vi "FPGA.vi"() -> ()   [LabVIEW 2020]
uses:
  <vilib>/Platform/TimedLoop/XDataNode/timing_clust.ctl
  <vilib>/Platform/TimedLoop/XDataNode/nitl_modes.ctl
  <vilib>/Platform/TimedLoop/XDataNode/wakeup.ctl
  <vilib>/rvi/Analysis/measure/FFT/simModelSupport/niFPGA FFT Sim Properties.ctl
  <vilib>/rvi/Analysis/measure/FFT/simModelSupport/niFPGA FFT Sim Types.ctl
  <vilib>/rvi/Analysis/measure/FFT/simModelSupport/niFpgaFFTSimArithmeticProperties.ctl
  <vilib>/rvi/Analysis/measure/FFT/simModelSupport/niFpgaFFTSimDfxp.ctl
  <vilib>/fxp/LVFixedPointQuantizationPolicyTypeDef.ctl
  <vilib>/rvi/DataTransferAndStorage/Container/Common/niFpgaContainerGetUniqueNameForEmu.vi
  <vilib>/rvi/DataTransferAndStorage/Container/Common/niFpgaContainerSetEmuInfo.vi
  <vilib>/rvi/eio/common/nirviEmuReportErrorAndStop.vi
  <vilib>/rvi/eio/common/nirviEmuTemplateMethod_errors.vi
  <vilib>/rvi/DataTransferAndStorage/Container/Common/niFpgaContainerExecOnDevCompGetState.vi
  <vilib>/rvi/Emulation/niFpgaEmulationIsFPGAContextNoSignature.vi
  <vilib>/rvi/Emulation/niFpgaSctlEmulationGetInTimedLoop.vi
  <vilib>/rvi/errors/niFpgaSetErrorForExecOnDevCompSimple.vi
  <vilib>/rvi/FIFO/Fifo_Resource/nirvififoEmulationSetSize.vi
  <vilib>/rvi/FIFO/Fifo_Resource/nirviFifoEmulationQueueMgr.vi
  <instcachedir>/0/nirviFifoEmulationQueueMgr_E5CAEC123FF24DC58D834DCA3CDAA9B5.lvgen/nirviFifoEmulationQueueMgr_E5CAEC123FF24DC58D834DCA3CDAA9B5_003.vi
  <vilib>/rvi/FIFO/Fifo_Resource/nirvififoEmulationDetermineInputValidOut.vi
  <vilib>/rvi/FIFO/Fifo_Resource/nirvififoEmulationCreateLock.vi
  <vilib>/rvi/Emulation/niFpgaProcessEmulError.vi
  <vilib>/rvi/FIFO/Fifo_Resource/nirvififoEmulationObtainLock.vi
  <vilib>/rvi/FIFO/Fifo_Resource/nirvififoEmulationReleaseLock.vi
  <vilib>/rvi/occurrence/nirviWaitOnOccurrenceBase.vi
  <vilib>/rvi/errors/nirviReportUnexpectedCaseInternalError.vi
  <vilib>/rvi/errors/nirviReportUnexpectedCaseInternalError (U32).vi
  <vilib>/Utility/error.llb/Clear Errors.vi
  <vilib>/rvi/interface/RandomDataEmulation/niFpgaRandomDataHandleErrors.vi
  <vilib>/rvi/Emulation/niFpgaEmulationReportErrorSimple.vi
  <vilib>/rvi/Emulation/niFpgaGetClockAttributes.vi
  <vilib>/rvi/Emulation/niFpgaCriticalErrorInLSC.vi
  <vilib>/rvi/Analysis/measure/FFT/simModelSupport/niFpgaFFTSimModelCore.vi
  <vilib>/rvi/LocalResourceManager/LocalResourceManager.xnode
  <vilib>/eio/EIONode/EIONode.xnode
  <vilib>/rvi/DataTransferAndStorage/Container/XNode/niFpgaContainer.xnode
  <vilib>/rvi/FIFO/Fifo_Resource/niFpgaFifoEmulationRefIn.vi
  <vilib>/Platform/TimedLoop/XDataNode/XDataNode.xnode
  <vilib>/rvi/interface/RandomDataEmulation/nirviRandomDataFpgaReadWriteTemplate.vi
  <vilib>/rvi/Analysis/measure/FFT/XNode/niFpgaFFT.xnode
  <vilib>/rvi/FXPMathLib/FxpInterpret/XNode/nifxpmath_Interpret.xnode
  <vilib>/Platform/TimedLoop/XDataNode/XDNodeRunTimeDep.lvlib
panel:
  in  "Rate (uSec)":u32 caption="Count(uSec)"
  out "Timed Out? FIFO out index 2":bool
  out "Timed Out? FIFO out IMG 2":bool
  out "Timed Out? FIFO out REAL 2":bool
  out "Timed Out? FIFO in IMG":bool
  out "Timed Out? FIFO in REAL":bool
  out "Timed Out? FIFO out REAL":bool
  out "Timed Out? FIFO out IMG":bool
  out "Timed Out? FIFO out index":bool
  in  "FFT loop iterations":i32
  in  "auto stop":bool
  in  "Loop number":i32
  out "AI Timed Out?":bool
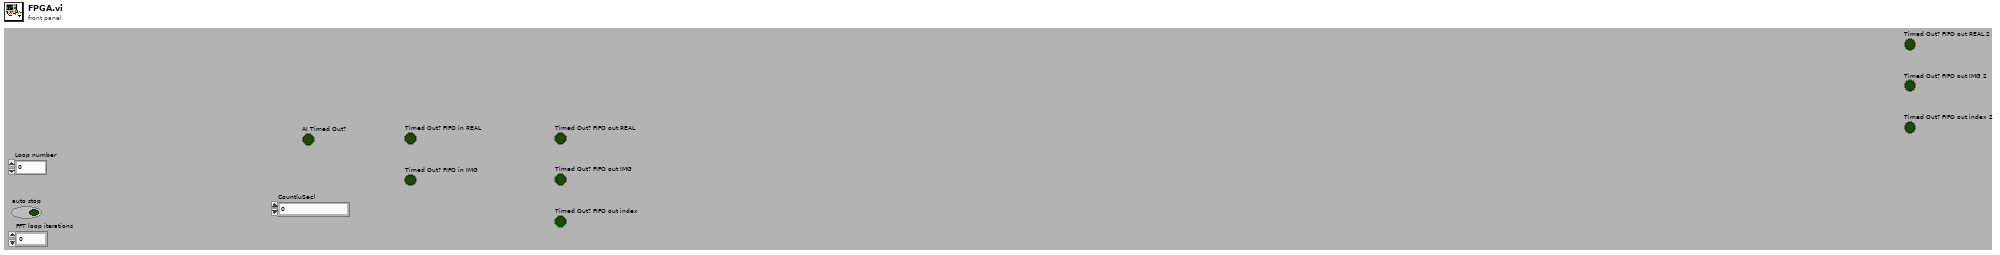
[diagram p1: front panel]
types:
  T1 = typedef "XDNodeRunTimeDep.lvlib/timing_clust.ctl" = cluster{"Expected End [f-1]":u64, "Actual End [f-1]":u64, "Finished Late? [f-1]":bool, "Expected End [i-1]":u64, "Actual End [i-1]":u64, "Finished Late? [i-1]":bool, "Expected Start [i]":u64, "Actual Start [i]":u64, "Expected Start [f]":u64, "Actual Start [f]":u64, "Source Name":string, "Structure Name":string, "Period":i64, "Deadline":i64, "Offset":i64, "Start":i64, "Priority":i32, "Timeout":i32, "Mode":T2, "Wakeup Reason":T3, "Error":errorcluster, "Source Type":string, "Secondary Source Type":string, "Global End Time":u64, "Global Start Time":u64, "Frame Duration":u64, "Iteration Duration":u64, "Assigned CPU":i32, "I/O Scan Engine Mode":u32}
  T2 = typedef "XDNodeRunTimeDep.lvlib/nitl_modes.ctl" = enum32{"No Change", "Process missed periods, maintain original phase", "Discard missed periods, maintain original phase", "Process missed periods, ignore original phase", "Discard missed periods, ignore original phase"}
  T3 = typedef "XDNodeRunTimeDep.lvlib/wakeup.ctl" = enum32{"Normal", "Aborted", "Asynchronous wakeup", "Timing source error", "Timed loop error", "Timeout"}
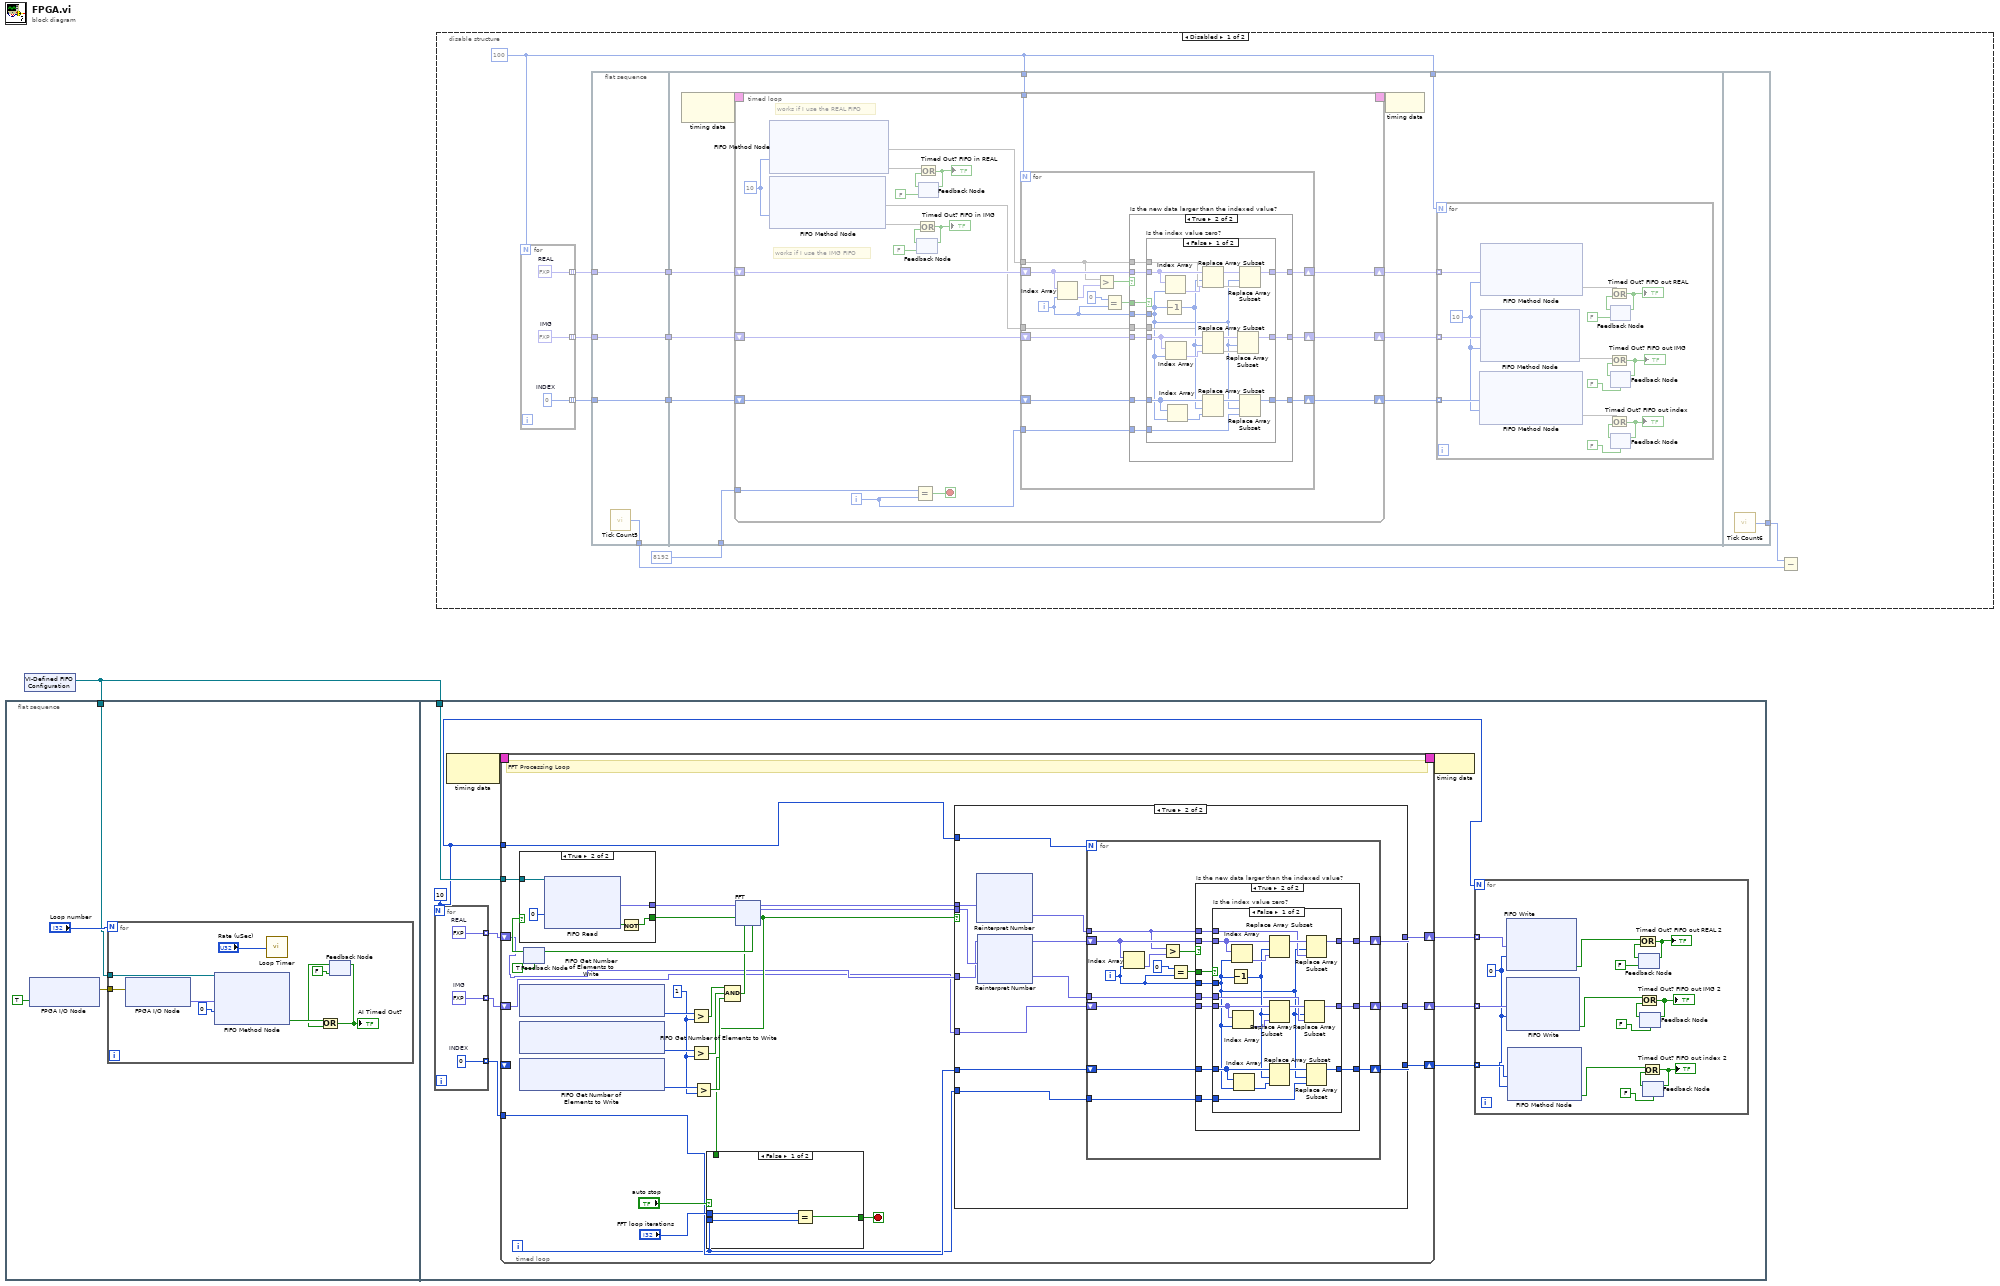
[diagram p0: block diagram]
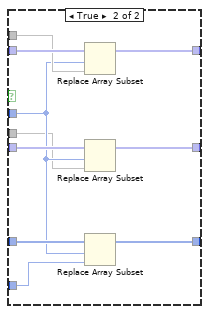
[diagram p3: hidden frame]
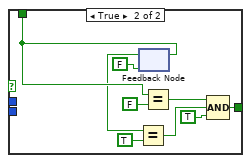
[diagram p5: hidden frame]
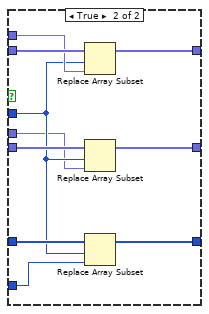
[diagram p8: hidden frame]
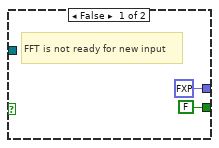
[diagram p9: hidden frame]
diagram:
  n1 = flat-sequence {
    tunnel: w1 -> [w4]
    tunnel: w1 -> [w22]
    frame #0 {
      n2 = xnode "FPGA I/O Node"("Mod1/Start"=TRUE) -> ("error out"=w2:errorcluster)  [unwired: 2 in, 1 out]
      n3 = for {
        N: "Loop number" -> [_]
        tunnel: w4 -> [w14]
        tunnel: w2 -> [w7]
        n4 = xnode "FPGA I/O Node"("error in"=w7) -> ("Mod1/AI0"=w8:fxp<+/-,24,7>)  [unwired: 1 in, 2 out]
        n5 = xnode ("FIFO Method Node")("Element"=w8, "Timeout"=0, "FIFO In"=w14) -> ("Timed Out?"=w12:bool)  [unwired: 1 in, 2 out]
        n6 = call "Loop Timer"("Count(uSec)"="Rate (uSec)") -> ()  [unwired: 1 out]
        n7 = feedback #1(FALSE) -> (w11:bool)
        n8 = Or(x=w12, y=w11) -> (x .or. y?=w10:bool)
        "AI Timed Out?" <- w10
        n9 = feedback-in #1(w10) -> ()
      }
    }
    frame #1 {
      w15 = 10
      n10 = for {
        N: w15 -> [_]
        tunnel: [w43] -> w21 mode=indexing
        tunnel: [w42] -> w19 mode=indexing
        tunnel: [w41] -> w20 mode=indexing
        w41 = fxp<+/-,32,21> 0.0  # IMG
        w42 = 0  # INDEX
        w43 = fxp<+/-,32,21> 0.0  # REAL
      }
      n11 = node-c288() -> (w24:T1)  [unwired: 1 in]
      n12 = timed-loop {
        timing: w24 -> [_]
        timing-out: [_] -> w23
        tunnel: w22 -> [w68]
        tunnel: w19 -> [w49]
        tunnel: w15 -> [w44]
        shift-right: [w45] -> w16
        shift-left: _ -> [_]
        shift-right: [w46] -> w18
        shift-left: w20 -> [w50]
        shift-right: [w47] -> w17
        shift-left: w21 -> [w51]
        i -> [w48]
        stop <- w56 stop-if-true
        w62 = u32 1 ("y")
        # "FFT Processing Loop"
        n13 = xnode ("FIFO Get Number of Elements to Write")() -> ("Number of Elements to Write"=w65:u32)  [unwired: 1 in, 1 out]
        n14 = xnode ("FIFO Get Number of Elements to Write")() -> ("Number of Elements to Write"=w64:u32)  [unwired: 1 in, 1 out]
        n15 = xnode ("FIFO Get Number of Elements to Write")() -> ("Number of Elements to Write"=w63:u32)  [unwired: 1 in, 1 out]
        n16 = feedback #2(TRUE ("ready for input")) -> (w71:bool)
        n17 = case shown="True" w71 {
          tunnel: [FALSE w185] -> w58
          tunnel: [fxp<+/-,16,5> 0.0 ("Element") w186] -> w70
          tunnel: w68 -> [_ w182]
          frame False {
            # "FFT is not ready for new input"
          }
          frame True {
            n18 = xnode ("FIFO Read")("Timeout"=0, "FIFO In"=w182) -> ("Element"=w186:fxp<+/-,24,7>, "Timed Out?"=w184:bool)  [unwired: 1 out]
            n19 = Not(x=w184) -> (.not. x?=w185:bool)
          }
        }
        n20 = Greater?(x=w65, y=w62) -> (0:w61:bool)
        n21 = Greater?(x=w64, y=w62) -> (0:w60:bool)
        n22 = Greater?(x=w63, y=w62) -> (0:w59:bool)
        n23 = Compound Arithmetic op=AND(w61, w60, w59) -> (w57:bool)
        n24 = xnode "FFT"("real data in"=w70, "input valid"=w58, "ready for output"=w57) -> ("ready for input"=w69:bool, "real data out"=w67:fxp<+/-,32,15>, "imaginary data out"=w55:fxp<+/-,32,15>, "output valid"=w52:bool)  [unwired: 2 in, 1 out]
        n25 = feedback-in #2(w69) -> ()
        n26 = case shown="False" "auto stop" {
          tunnel: w52 -> [_ w82]
          tunnel: [w72 w75] -> w56
          tunnel: w48 -> [w74 _]
          tunnel: "FFT loop iterations" -> [w73 _]
          frame False {
            n27 = Equal?(x=w73, y=w74) -> (x = y?=w72:bool)
          }
          frame True {
            n28 = feedback #3(FALSE) -> (w79:bool)
            n29 = Equal?(x=w79, y=TRUE) -> (x = y?=w77:bool)
            n30 = feedback-in #3(w82) -> ()
            n31 = Equal?(x=w82, y=FALSE) -> (x = y?=w78:bool)
            n32 = Compound Arithmetic op=AND(w78, w77, TRUE ("value")) -> (w75:bool)
          }
        }
        n33 = case shown="True" w52 {
          tunnel: w67 -> [_ w124]
          tunnel: w55 -> [_ w123]
          tunnel: w51 -> [w112 w120]
          tunnel: w50 -> [w111 w119]
          tunnel: w49 -> [w110 w118]
          tunnel: w48 -> [_ w117]
          tunnel: [w112 w116] -> w47
          tunnel: [w111 w115] -> w46
          tunnel: [w110 w114] -> w45
          tunnel: w44 -> [_ w113]
          frame False {
          }
          frame True {
            n34 = xnode "Reinterpret Number"("x"=w124) -> ("y"=w122:fxp<+/-,32,21>)
            n35 = xnode "Reinterpret Number"("x"=w123) -> ("y"=w121:fxp<+/-,32,21>)
            n36 = for {
              N: w113 -> [_]
              tunnel: w122 -> [w135]
              shift-right: [w134] -> w116
              shift-left: w120 -> [w136]
              tunnel: w117 -> [w132]
              shift-right: [w130] -> w114
              shift-left: w118 -> [w131]
              shift-right: [w127] -> w115
              shift-left: w119 -> [w126]
              tunnel: w121 -> [w125]
              i -> [w133]
              n37 = Index Array(array=w136, index=w133) -> (element=w138:fxp<+/-,32,21>)
              n38 = Greater?(x=w135, y=w138) -> (0:w137:bool)
              n39 = Equal?(x=0, y=w133) -> (x = y?=w128:bool)
              n40 = case "Is the new data larger than the indexed value?" shown="True" w137 {
                tunnel: w136 -> [w141 w151]
                tunnel: w128 -> [_ w152]
                tunnel: w135 -> [_ w150]
                tunnel: w133 -> [_ w149]
                tunnel: [w141 w148] -> w134
                tunnel: w132 -> [_ w147]
                tunnel: w131 -> [w140 w146]
                tunnel: [w140 w145] -> w130
                tunnel: [w139 w144] -> w127
                tunnel: w126 -> [w139 w143]
                tunnel: w125 -> [_ w142]
                frame False {
                }
                frame True {
                  n41 = case "Is the index value zero?" shown="False" w152 {
                    tunnel: w151 -> [w169 w179]
                    tunnel: w150 -> [w166 w178]
                    tunnel: w149 -> [w153 w172]
                    tunnel: [w165 w177] -> w148
                    tunnel: w147 -> [w160 w176]
                    tunnel: w146 -> [w162 w175]
                    tunnel: [w161 w174] -> w145
                    tunnel: [w155 w170] -> w144
                    tunnel: w143 -> [w159 w173]
                    tunnel: w142 -> [w154 w171]
                    frame False {
                      n42 = Decrement(x=w153) -> (x-1=w157:i32)
                      n43 = Index Array(array=w169, index=w153) -> (element=w168:fxp<+/-,32,21>)
                      n44 = Index Array(array=w159, index=w153) -> (element=w158:fxp<+/-,32,21>)
                      n45 = Index Array(array=w162, index=w153) -> (element=w164:i32)
                      n46 = Replace Array Subset(array=w169, new element=w168, index=w157) -> (w167:fxp<+/-,32,21>[])
                      n47 = Replace Array Subset(array=w159, new element=w158, index=w157) -> (w156:fxp<+/-,32,21>[])
                      n48 = Replace Array Subset(array=w162, new element=w164, index=w157) -> (w163:i32[])
                      n49 = Replace Array Subset(array=w156, new element=w154, index=w153) -> (w155:fxp<+/-,32,21>[])
                      n50 = Replace Array Subset(array=w167, new element=w166, index=w153) -> (w165:fxp<+/-,32,21>[])
                      n51 = Replace Array Subset(array=w163, new element=w160, index=w153) -> (w161:i32[])
                    }
                    frame True {
                      n52 = Replace Array Subset(array=w179, new element=w178, index=w172) -> (w177:fxp<+/-,32,21>[])
                      n53 = Replace Array Subset(array=w173, new element=w171, index=w172) -> (w170:fxp<+/-,32,21>[])
                      n54 = Replace Array Subset(array=w175, new element=w176, index=w172) -> (w174:i32[])
                    }
                  }
                }
              }
            }
          }
        }
      }
      n55 = node-c288(w23) -> ()
      n56 = for {
        N: w15 -> [_]
        tunnel: w18 -> [w40] mode=indexing
        tunnel: w17 -> [w39] mode=indexing
        tunnel: w16 -> [w29] mode=indexing
        w28 = 0 ("Timeout")
        n57 = xnode ("FIFO Write")("Element"=w39, "Timeout"=w28) -> ("Timed Out?"=w25:bool)  [unwired: 1 in, 1 out]
        n58 = xnode ("FIFO Write")("Element"=w40, "Timeout"=w28) -> ("Timed Out?"=w26:bool)  [unwired: 1 in, 1 out]
        n59 = xnode ("FIFO Method Node")("Element"=w29, "Timeout"=w28) -> ("Timed Out?"=w27:bool)  [unwired: 1 in, 1 out]
        n60 = feedback #4(FALSE) -> (w36:bool)
        n61 = Or(x=w25, y=w36) -> (x .or. y?=w37:bool)
        "Timed Out? FIFO out REAL 2" <- w37
        n62 = feedback-in #4(w37) -> ()
        n63 = feedback #5(FALSE) -> (w35:bool)
        n64 = Or(x=w26, y=w35) -> (x .or. y?=w34:bool)
        "Timed Out? FIFO out IMG 2" <- w34
        n65 = feedback-in #5(w34) -> ()
        n66 = feedback #6(FALSE) -> (w32:bool)
        n67 = Or(x=w27, y=w32) -> (x .or. y?=w31:bool)
        "Timed Out? FIFO out index 2" <- w31
        n68 = feedback-in #6(w31) -> ()
      }
    }
  }
  n69 = xnode "VI-Defined FIFO Configuration"() -> ("FIFO Out"=w1:refnum<k21>)
  n70 = disable-structure shown="Disabled" {
    frame Disabled {
      w192 = 100
      n71 = for {
        N: w192 -> [_]
        tunnel: [w203] -> w194 mode=indexing
        tunnel: [w202] -> w195 mode=indexing
        tunnel: [w201] -> w191 mode=indexing
        w201 = fxp<+/-,32,21> 0.0  # IMG
        w202 = 0  # INDEX
        w203 = fxp<+/-,32,21> 0.0  # REAL
      }
      n72 = flat-sequence {
        tunnel: [w207] -> w196
        tunnel: [w206] -> w200
        tunnel: w195 -> [w206]
        tunnel: [w205] -> w199
        tunnel: w194 -> [w205]
        tunnel: [w204] -> w198
        tunnel: w191 -> [w204]
        tunnel: w200 -> [w218]
        tunnel: w199 -> [w217]
        tunnel: 8192 ("samples") -> [w215]
        tunnel: w192 -> [w216]
        tunnel: w192 -> [w212]
        tunnel: w198 -> [w208]
        tunnel: [w315] -> w197
        frame #0 {
          n73 = call "Tick Count5"() -> ("Tick Count(uSec)"=w207:u32)
        }
        frame #1 {
          n74 = node-c288() -> (w214:T1)  [unwired: 1 in]
          n75 = timed-loop {
            shift-right: [w254] -> w210
            shift-left: w217 -> [w255]
            shift-right: [w253] -> w211
            shift-left: w218 -> [w252]
            tunnel: w216 -> [w251]
            tunnel: w215 -> [w249]
            timing: w214 -> [_]
            timing-out: [_] -> w213
            shift-right: [w247] -> w209
            shift-left: w208 -> [w246]
            i -> [w250]
            stop <- w248 stop-if-true
            w245 = 10 ("Timeout")
            # "works if I use the REAL FIFO"
            # "works if I use the IMG FIFO"
            n76 = xnode ("FIFO Method Node")("Timeout"=w245) -> ("Element"=w243, "Timed Out?"=w235)  [unwired: 1 in, 1 out]
            n77 = xnode ("FIFO Method Node")("Timeout"=w245) -> ("Element"=w244, "Timed Out?"=w239)  [unwired: 1 in, 1 out]
            n78 = Equal?(x=w249, y=w250) -> (x = y?=w248:bool)
            n79 = feedback #7(FALSE) -> (w240:bool)
            n80 = Or(x=w239, y=w240) -> (x .or. y?=w241:bool)
            "Timed Out? FIFO in IMG" <- w241
            n81 = feedback-in #7(w241) -> ()
            n82 = feedback #8(FALSE) -> (w236:bool)
            n83 = Or(x=w235, y=w236) -> (x .or. y?=w237:bool)
            "Timed Out? FIFO in REAL" <- w237
            n84 = feedback-in #8(w237) -> ()
            n85 = for {
              N: w251 -> [_]
              tunnel: w243 -> [w266]
              shift-right: [w265] -> w254
              shift-left: w255 -> [w267]
              tunnel: w250 -> [w263]
              shift-right: [w261] -> w253
              shift-left: w252 -> [w262]
              shift-right: [w258] -> w247
              shift-left: w246 -> [w257]
              tunnel: w244 -> [w256]
              i -> [w264]
              n86 = Index Array(array=w267, index=w264) -> (element=w269:fxp<+/-,32,21>)
              n87 = Greater?(x=w266, y=w269) -> (0:w268:bool)
              n88 = Equal?(x=0, y=w264) -> (x = y?=w259:bool)
              n89 = case "Is the new data larger than the indexed value?" shown="True" w268 {
                tunnel: w267 -> [w272 w282]
                tunnel: w259 -> [_ w283]
                tunnel: w266 -> [_ w281]
                tunnel: w264 -> [_ w280]
                tunnel: [w272 w279] -> w265
                tunnel: w263 -> [_ w278]
                tunnel: w262 -> [w271 w277]
                tunnel: [w271 w276] -> w261
                tunnel: [w270 w275] -> w258
                tunnel: w257 -> [w270 w274]
                tunnel: w256 -> [_ w273]
                frame False {
                }
                frame True {
                  n90 = case "Is the index value zero?" shown="False" w283 {
                    tunnel: w282 -> [w300 w310]
                    tunnel: w281 -> [w297 w309]
                    tunnel: w280 -> [w284 w303]
                    tunnel: [w296 w308] -> w279
                    tunnel: w278 -> [w291 w307]
                    tunnel: w277 -> [w293 w306]
                    tunnel: [w292 w305] -> w276
                    tunnel: [w286 w301] -> w275
                    tunnel: w274 -> [w290 w304]
                    tunnel: w273 -> [w285 w302]
                    frame False {
                      n91 = Decrement(x=w284) -> (x-1=w288:i32)
                      n92 = Index Array(array=w300, index=w284) -> (element=w299:fxp<+/-,32,21>)
                      n93 = Index Array(array=w290, index=w284) -> (element=w289:fxp<+/-,32,21>)
                      n94 = Index Array(array=w293, index=w284) -> (element=w295:i32)
                      n95 = Replace Array Subset(array=w300, new element=w299, index=w288) -> (w298:fxp<+/-,32,21>[])
                      n96 = Replace Array Subset(array=w290, new element=w289, index=w288) -> (w287:fxp<+/-,32,21>[])
                      n97 = Replace Array Subset(array=w293, new element=w295, index=w288) -> (w294:i32[])
                      n98 = Replace Array Subset(array=w287, new element=w285, index=w284) -> (w286:fxp<+/-,32,21>[])
                      n99 = Replace Array Subset(array=w298, new element=w297, index=w284) -> (w296:fxp<+/-,32,21>[])
                      n100 = Replace Array Subset(array=w294, new element=w291, index=w284) -> (w292:i32[])
                    }
                    frame True {
                      n101 = Replace Array Subset(array=w310, new element=w309, index=w303) -> (w308:fxp<+/-,32,21>[])
                      n102 = Replace Array Subset(array=w304, new element=w302, index=w303) -> (w301:fxp<+/-,32,21>[])
                      n103 = Replace Array Subset(array=w306, new element=w307, index=w303) -> (w305:i32[])
                    }
                  }
                }
              }
            }
          }
          n104 = node-c288(w213) -> ()
          n105 = for {
            N: w212 -> [_]
            tunnel: w211 -> [w234] mode=indexing
            tunnel: w210 -> [w233] mode=indexing
            tunnel: w209 -> [w232] mode=indexing
            w231 = 10 ("Timeout")
            n106 = xnode ("FIFO Method Node")("Element"=w234, "Timeout"=w231) -> ("Timed Out?"=w219)  [unwired: 1 in, 1 out]
            n107 = xnode ("FIFO Method Node")("Element"=w233, "Timeout"=w231) -> ("Timed Out?"=w227)  [unwired: 1 in, 1 out]
            n108 = xnode ("FIFO Method Node")("Element"=w232, "Timeout"=w231) -> ("Timed Out?"=w223)  [unwired: 1 in, 1 out]
            n109 = feedback #9(FALSE) -> (w228:bool)
            n110 = Or(x=w227, y=w228) -> (x .or. y?=w229:bool)
            "Timed Out? FIFO out REAL" <- w229
            n111 = feedback-in #9(w229) -> ()
            n112 = feedback #10(FALSE) -> (w226:bool)
            n113 = Or(x=w223, y=w226) -> (x .or. y?=w225:bool)
            "Timed Out? FIFO out IMG" <- w225
            n114 = feedback-in #10(w225) -> ()
            n115 = feedback #11(FALSE) -> (w222:bool)
            n116 = Or(x=w219, y=w222) -> (x .or. y?=w221:bool)
            "Timed Out? FIFO out index" <- w221
            n117 = feedback-in #11(w221) -> ()
          }
        }
        frame #2 {
          n118 = call "Tick Count6"() -> ("Tick Count(uSec)"=w315:u32)
        }
      }
      n119 = Subtract(x=w197, y=w196) -> ()  [unwired: 1 out]
    }
    frame Enabled {
    }
  }
